vi "Get Time.vi"(9 "Date":string, 10 "# of rows":i32, 11 "Data row":string[][](array[string])) -> (3 "Time array":timestamp[](array[timestamp]))   [LabVIEW 2014]
panel:
  out "Numeric":i32
  out "hour":string
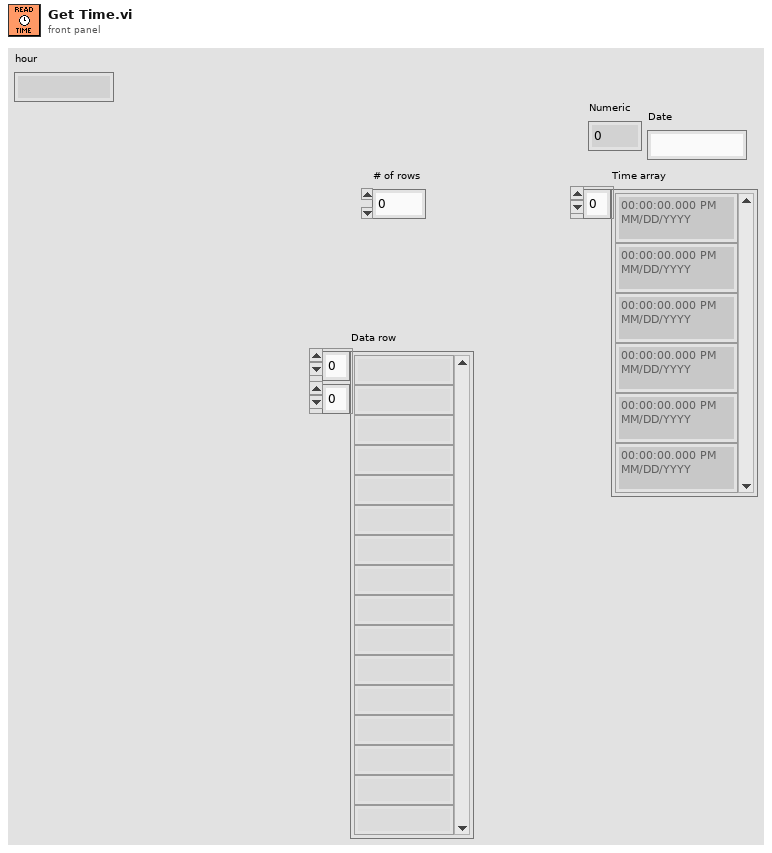
[diagram p1: front panel]
types:
  T1 = typedef "LVDateTimeRec.ctl" = cluster{"fractional second":dbl, "second":i32, "minute":i32, "hour":i32, "day of month":i32, "month":i32, "year":i32, "day of week":i32, "day of year":i32, "DST":i32}
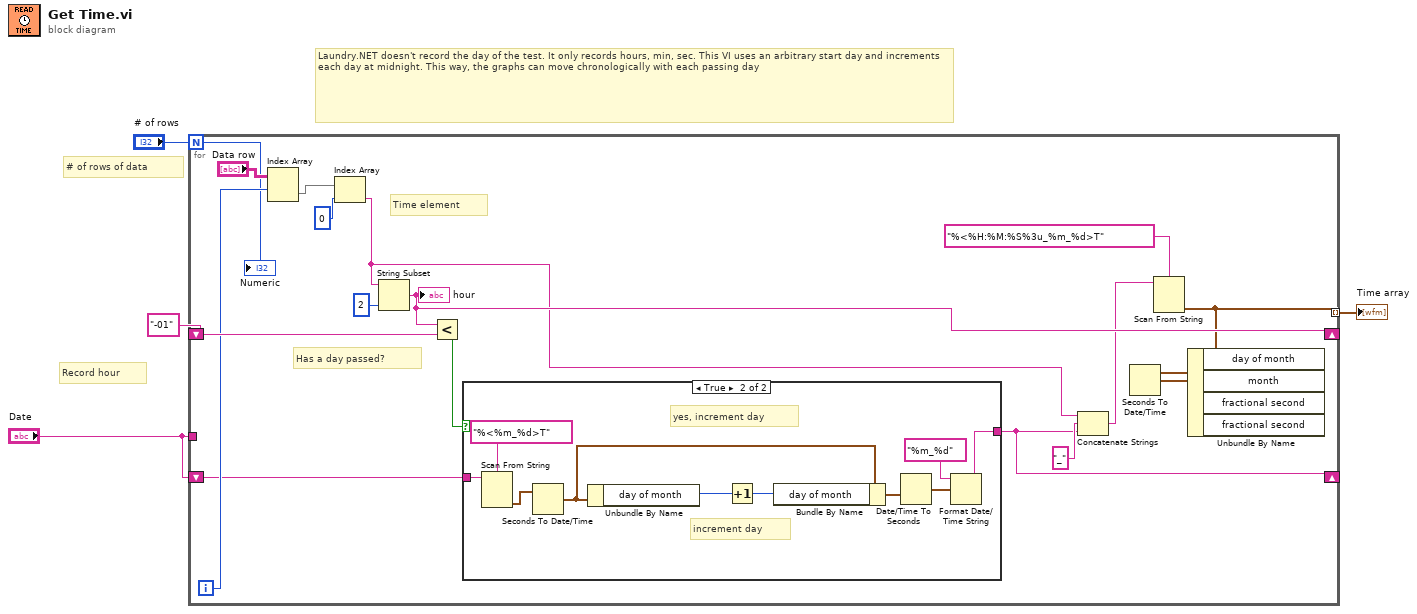
[diagram p0: block diagram]
diagram:
  # "Record hour"
  # "Laundry.NET doesn't record the day of the test. It only records hours, min, sec. This VI uses an arbitrary start day and increments each day at midnight. This way, the graphs can move chronologically with each passing day"
  # "# of rows of data"
  n1 = for {
    N: "# of rows" -> [w10]
    shift-right: [w17] -> _
    shift-left: "-01" ("String") -> [w16]
    tunnel: [w9] -> w3 mode=indexing
    tunnel: "Date" -> [_]
    shift-right: [w5] -> _
    shift-left: "Date" -> [w6]
    i -> [w13]
    # "Time element"
    # "Has a day passed?"
    n2 = Index Array(array="Data row", index (row)=w13) -> (element=w15:string[])  [unwired: 1 in]
    n3 = Index Array(array=w15, index=0) -> (element=w12:string)
    n4 = String Subset(string=w12, length (rest)=2 ("length (rest)")) -> (substring=w17:string)  [unwired: 1 in]
    "hour" <- w17
    n5 = Less?(x=w17, y=w16) -> (x < y?=w19:bool)
    n6 = case shown="True" w19 {
      tunnel: [w22 w23] -> w5
      tunnel: w6 -> [w22 w24]
      frame False {
        # "No, same day"
      }
      frame True {
        # "increment day"
        # "yes, increment day"
        n7 = Scan From String(format string="%<%m_%d>T", input string=w24) -> (output 1=w31:timestamp)  [unwired: 3 in, 3 out]
        n8 = Seconds To Date/Time(time stamp (now)=w31) -> (date time rec=w29:T1)  [unwired: 1 in]
        n9 = Unbundle By Name(w29) -> ("day of month"=w30:i32)
        n10 = Increment(x=w30) -> (x+1=w28:i32)
        n11 = Bundle By Name(cluster=w29, "day of month"=w28) -> (w27:T1)
        n12 = Date/Time To Seconds(2:w27) -> (0:w26:timestamp)  [unwired: 1 in]
        n13 = Format Date/Time String(time format string (%c)="%m_%d", seconds (now)=w26) -> (date/time string=w23:string)  [unwired: 1 in]
      }
    }
    n14 = Concatenate Strings(w12, "_" ("string"), w5) -> (w11:string)
    n15 = Scan From String(format string="%<%H:%M:%S%3u_%m_%d>T", input string=w11) -> (output 1=w9:timestamp)  [unwired: 3 in, 3 out]
    n16 = Seconds To Date/Time(time stamp (now)=w9) -> (date time rec=w8:T1)  [unwired: 1 in]
    n17 = Unbundle By Name(w8) -> ()  [unwired: 4 out]
    "Numeric" <- w10
  }
  "Time array" <- w3
